vi "Package_MFC_Data.vi"(8 "Error in":errorcluster, 10 "MFC Data In":T1, 11 "MFC ID":string) -> (2 "String Array Output":string[](array[string]))   [LabVIEW 2019]
panel:
  # "Totalizer Timer"
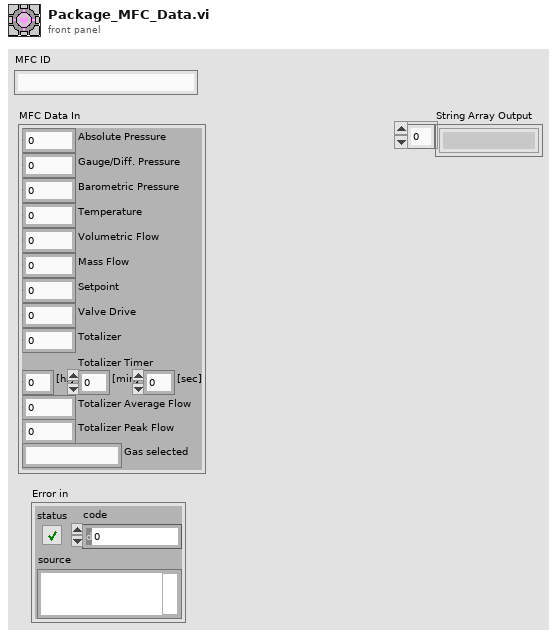
[diagram p1: front panel]
types:
  T1 = cluster{"Absolute Pressure":dbl, "Gauge/Diff. Pressure":dbl, "Barometric Pressure":dbl, "Temperature":dbl, "Volumetric Flow":dbl, "Mass Flow":dbl, "Setpoint":dbl, "Valve Drive":dbl, "Totalizer":dbl, "[hr]":dbl, "[min]":dbl, "[sec]":dbl, "Totalizer Average Flow":dbl, "Totalizer Peak Flow":dbl, "Gas selected":string}
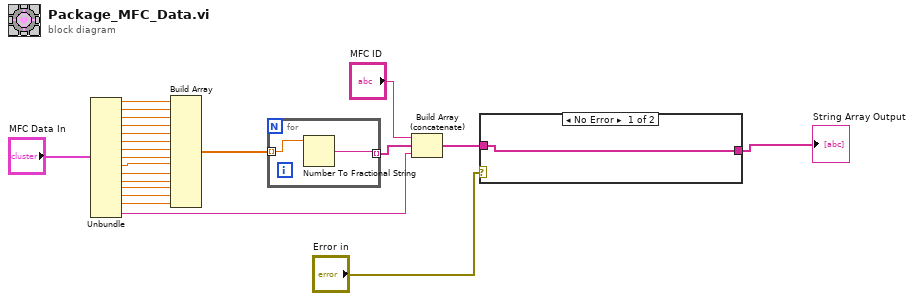
[diagram p0: block diagram]
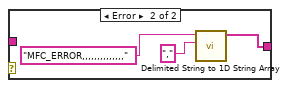
[diagram p2: hidden frame]
diagram:
  n1 = Unbundle("MFC Data In") -> ("Absolute Pressure"=w21:dbl, "Gauge/Diff. Pressure"=w8:dbl, "Barometric Pressure"=w9:dbl, "Temperature"=w10:dbl, "Volumetric Flow"=w11:dbl, "Mass Flow"=w12:dbl, "Setpoint"=w13:dbl, "Valve Drive"=w14:dbl, "Totalizer"=w15:dbl, "[hr]"=w16:dbl, "[min]"=w17:dbl, "[sec]"=w18:dbl, "Totalizer Average Flow"=w19:dbl, "Totalizer Peak Flow"=w20:dbl, "Gas selected"=w5:string)
  n2 = Build Array(w21, w8, w9, w10, w11, w12, w13, w14, w15, w16, w17, w18, w19, w20) -> (w7:dbl[])
  n3 = for {
    tunnel: w7 -> [w24] mode=indexing
    tunnel: [w23] -> w6 mode=indexing
    n4 = Number To Fractional String(number=w24) -> (F-format string=w23:string)  [unwired: 3 in]
  }
  n5 = Build Array (concatenate)("MFC ID", w6, w5) -> (w2:string[])
  n6 = case shown="No Error" "Error in" {
    tunnel: w2 -> [w25 _]
    tunnel: [w25 w26] -> w1
    frame No Error {
    }
    frame Error {
      n7 = call <vilib>:"Delimited String to 1D String Array.vi"("delimiter"=",", "delimited string"="MFC_ERROR,,,,,,,,,,,,,,") -> ("string array"=w26:string[])  [unwired: 9 in]
    }
  }
  "String Array Output" <- w1
